vi "Subtract Vec3d.vi"(8 "error in (no error)":errorcluster, 10 "Vec3d in 2":refnum<class "Vec3d Class.lvclass">, 11 "Vec3d in 1":refnum<class "Vec3d Class.lvclass">) -> (0 "error out":errorcluster, 3 "Vec3d Class out":refnum<class "Vec3d Class.lvclass">)   [LabVIEW 2011, in "Vec3d Class.lvclass"]
uses:
  Vec3d Class.lvclass
  Vec3d Class.lvclass/Vec3d Class.ctl
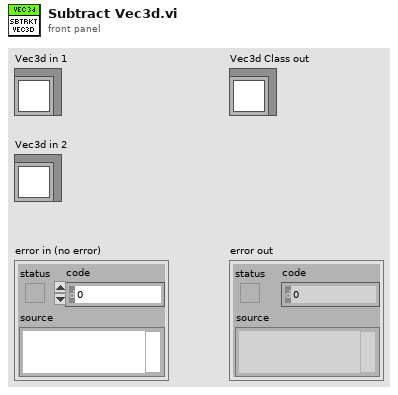
[diagram p1: front panel]
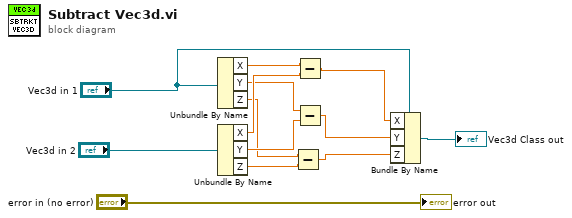
[diagram p0: block diagram]
diagram:
  n1 = Unbundle By Name("Vec3d in 1") -> ("X"=w11:dbl, "Y"=w8:dbl, "Z"=w6:dbl)
  n2 = Unbundle By Name("Vec3d in 2") -> ("X"=w10:dbl, "Y"=w7:dbl, "Z"=w5:dbl)
  n3 = Subtract(x=w6, y=w5) -> (x-y=w3:dbl)
  n4 = Subtract(x=w11, y=w10) -> (x-y=w9:dbl)
  n5 = Subtract(x=w8, y=w7) -> (x-y=w4:dbl)
  n6 = Bundle By Name(cluster="Vec3d in 1", "X"=w9, "Y"=w4, "Z"=w3) -> (→"Vec3d Class out":refnum<class "Vec3d Class.lvclass">)
  "error out" <- "error in (no error)"
